vi "wa32 ReadFile.vi"(8 "error in":errorcluster, 10 "bytes to read (0)":i32, 11 "handle":i32) -> (0 "error out":errorcluster, 1 "read bytes":u32, 2 "read data":u8[](array[numeric]), 3 "handle out":i32, 4 "read string":string)   [LabVIEW 2020]
doc: "WinAPI ReadFile() wrapper. For reading opened handle (files, devices, pipes, ...)."
uses:
  <vilib>/Utility/error.llb/Error Cluster From Error Code.vi
  <vilib>/ErrorRing/Error Ring.xnode
  kernel32.dll
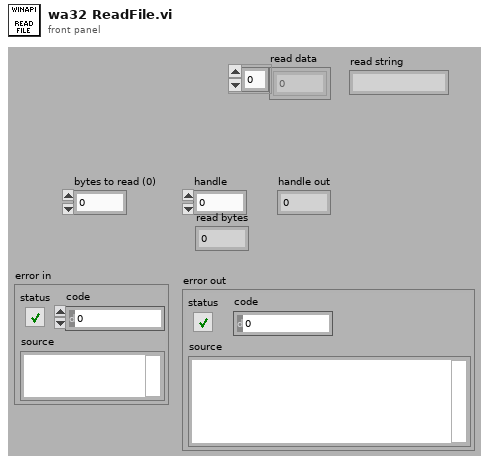
[diagram p1: front panel]
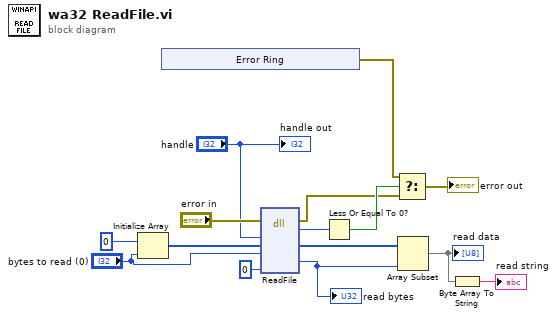
[diagram p0: block diagram]
diagram:
  n1 = Initialize Array(u8 0, "bytes to read (0)") -> (w7:u8[])
  n2 = xnode "Error Ring"() -> ("error out"=w10:errorcluster)
  n3 = dll-call lib="kernel32.dll" fn="ReadFile"(error in="error in", "handle"="handle", "data"=w7, "toRead"="bytes to read (0)", "overlapped"=0) -> (error out=w12:errorcluster, "errout"=w14:i32, "data"=w4:u8[], "read"=w3:u32)  [unwired: 6 in, 1 out]
  "read bytes" <- w3
  n4 = Less Or Equal To 0?(x=w14) -> (x <= 0?=w13:bool)
  n5 = Select(t=w10, s=w13, f=w12) -> (s? t:f=→"error out":errorcluster)
  n6 = Array Subset(array=w4, length=w3) -> (w2:u8[])  [unwired: 1 in]
  "read data" <- w2
  n7 = Byte Array To String(unsigned byte array=w2) -> (string=→"read string":string)
  "handle out" <- "handle"
